vi "edittest Sequence FIELDS.vi"(7 "Template Keys In (empty)":T1, 8 "error in (no error)":errorcluster, 9 "fSpartanSetsSN":bool, 10 "Sequence Id (\"\")":string, 11 "Connection Refnum":T2) -> (0 "error out":errorcluster, 3 "Connection Refnum":T2, 5 "Template Keys Out":T1)   [LabVIEW 2011]
uses:
  Summitek EXT/ODBC/SQL Controls/Connection Refnum.ctl
  ITK EXT/utils/keyedarr.llb/Keyed Array.ctl
  ITK EXT/utils/strutil.llb/Case Matching.ctl
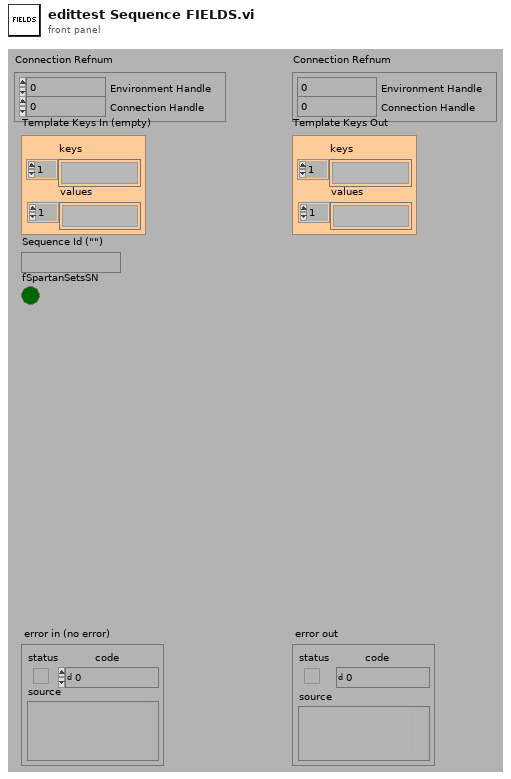
[diagram p1: front panel]
types:
  T1 = typedef "Keyed Array.ctl" = cluster{"keys":string[], "values":string[]}
  T2 = typedef "Connection Refnum.ctl" = cluster{"Environment Handle":i32, "Connection Handle":i32}
  T3 = typedef "Case Matching.ctl" = enum16{"a != A", "a == A", "system"}
  T4 = typedef "Field Record.ctl" = cluster{"ixField":i32, "iSequenceOrder":i32, "sxFieldId":string, "sxSequenceId":string, "sDisplayName":string, "sValue":string, "sUnits":string, "nDataType":T5, "nNextItem":T6, "fSystem":bool, "fSystemValue":bool, "fRequired":bool, "fSetAtTest":bool, "fTestField":bool, "fDeleted":bool, "fIndexed":bool, "fFreeList":bool}
  T5 = typedef "Field DataTypes.ctl" = enum32{"text", "numeric", "list", "timestamp", "boolean"}
  T6 = typedef "Field NextItem.ctl" = enum32{"Reset", "Retain", "Auto-Increment"}
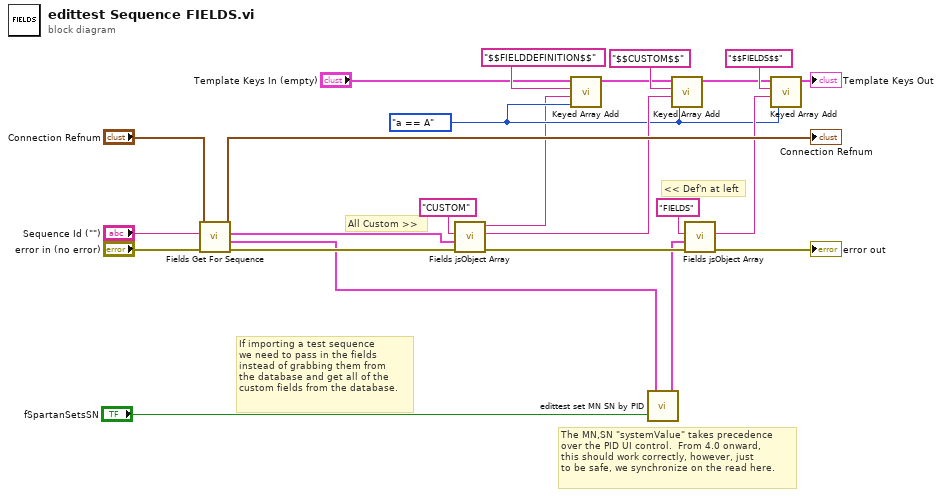
[diagram p0: block diagram]
diagram:
  w3 = Case_Matching."a == A" ("case matching (sensitive)")
  # "<< Def'n at left"
  # "All Custom >>"
  # "If importing a test sequence\nwe need to pass in the fields\ninstead of grabbing them from\nthe database and get all of the\ncustom fields from the database."
  # "The MN,SN \"systemValue\" takes precedence\nover the PID UI control.  From 4.0 onward,\nthis should work correctly, however, just\nto be safe, we synchronize on the read here."
  n1 = call "Fields Get For Sequence.vi"("error in (no error)"="error in (no error)", "sxSequenceId (\"\")"="Sequence Id (\"\")", "Connection Refnum"="Connection Refnum") -> ("error out"=w21:errorcluster, "Current Sequence Fields"=w1:T4[], "All Custom Fields"=w19:T4[], "Connection Refnum"=→"Connection Refnum":T2)  [unwired: 5 out]
  n2 = call "Fields jsObject Array.vi"("error in (no error)"=w21, "FIELDS (none)"=w19, "Fields jsObject Array Name (\"FIELDS\")"="CUSTOM") -> ("error out"=w15:errorcluster, "Fields jsObject Array"=w6:string, "Field jsObject Definition"=w2:string)  [unwired: 1 in, 5 out]
  n3 = call "Keyed Array Add.vi"("case matching (sensitive)"=w3, "value"=w2, "key"="$$FIELDDEFINITION$$", "array in"="Template Keys In (empty)") -> ("array out"=w4:T1)  [unwired: 3 out]
  n4 = call "edittest set MN SN by PID.vi"("fSpartanSetsSN"="fSpartanSetsSN", "FIELDS (empty)"=w1) -> ("FIELDS out"=w13:T4[])  [unwired: 1 out]
  n5 = call "Keyed Array Add.vi"("case matching (sensitive)"=w3, "value"=w6, "key"="$$CUSTOM$$", "array in"=w4) -> ("array out"=w16:T1)  [unwired: 3 out]
  n6 = call "Fields jsObject Array.vi"("error in (no error)"=w15, "FIELDS (none)"=w13, "Fields jsObject Array Name (\"FIELDS\")"="FIELDS") -> ("error out"=→"error out":errorcluster, "Fields jsObject Array"=w7:string)  [unwired: 1 in, 6 out]
  n7 = call "Keyed Array Add.vi"("case matching (sensitive)"=w3, "value"=w7, "key"="$$FIELDS$$", "array in"=w16) -> ("array out"=→"Template Keys Out":T1)  [unwired: 3 out]
